vi "set sync out settings.vi"(8 "error in (no error)":errorcluster, 10 "sync_out_settings":T1, 11 "id":i32) -> (0 "error out":errorcluster, 3 "function return":i32)   [LabVIEW 2020, in "libximc.lvlib"]
doc: "result_t XIMC_API set_sync_out_settings (device_t id, const sync_out_settings_t* sync_out_settings);"
uses:
  libximc.lvlib
  libximc.dll
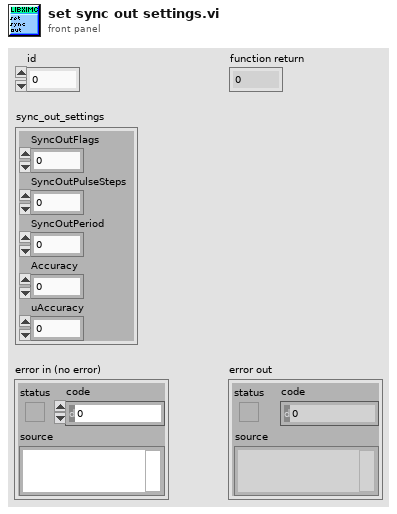
[diagram p1: front panel]
types:
  T1 = cluster{"SyncOutFlags":u32, "SyncOutPulseSteps":u32, "SyncOutPeriod":u32, "Accuracy":u32, "uAccuracy":u32}
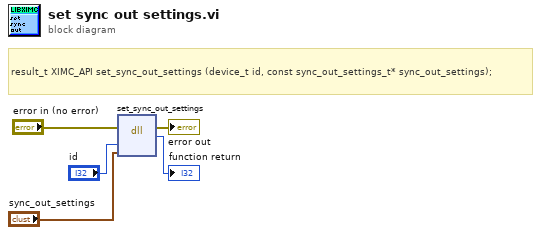
[diagram p0: block diagram]
diagram:
  # "result_t XIMC_API set_sync_out_settings (device_t id, const sync_out_settings_t* sync_out_settings);"
  n1 = dll-call lib="E:/Norway Project/All Hardware/New Microscope/LabVIEW/Stage/libximc.*" fn="set_sync_out_settings"(error in="error in (no error)", "id"="id", "sync_out_settings"="sync_out_settings") -> (error out=→"error out":errorcluster, →"function return":i32)  [unwired: 4 in, 1 out]
